vi "TSM Relay Control.vi"(0 "Relay TSM in":T1, 2 "Settling Time (s)":dbl, 5 "Relay Action":T3=21 items=["Open Relay"=20, "Close Relay"=21], 11 "error in":errorcluster) -> (15 "error out":errorcluster)   [LabVIEW 2020]
doc: "Performs the specified relay action on all specified relays."
uses:
  <vilib>/NI_TestStand_SemiconductorModule/NI_TestStand_Semiconductor_Module.lvlibp/1abvi3w/instr.lib/niSwitch/niswitch.llb/niSwitch Relay Action.ctl
  Pin Map/TSM Relay.ctl
  <vilib>/NI_TestStand_SemiconductorModule/NI_TestStand_Semiconductor_Module.lvlibp/PinMap/General/SemiconductorModuleContext.ctl
  <vilib>/NI_TestStand_SemiconductorModule/NI_TestStand_Semiconductor_Module.lvlibp/PinMap/Relay Driver/ControlRelaysSingleAction.vi
  <vilib>/NI_TestStand_SemiconductorModule/NI_TestStand_Semiconductor_Module.lvlibp
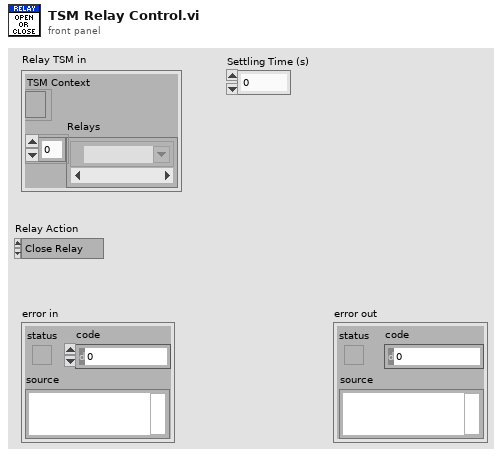
[diagram p1: front panel]
types:
  T1 = typedef "TSM Relay.ctl" = cluster{"TSM Context":T2, "Relays":tag[]}
  T2 = typedef "NI_TestStand_Semiconductor_Module.lvlibp/SemiconductorModuleContext.ctl" = refnum<k7>
  T3 = typedef "NI_TestStand_Semiconductor_Module.lvlibp/niSwitch Relay Action.ctl" = i32
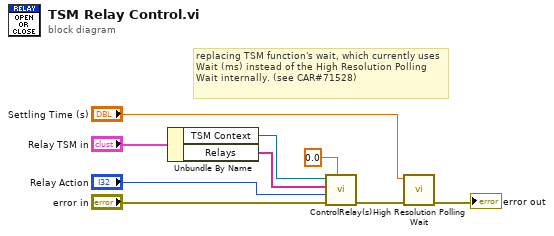
[diagram p0: block diagram]
diagram:
  # "replacing TSM function's wait, which currently uses Wait (ms) instead of the High Resolution Polling Wait internally. (see CAR#71528)"
  n1 = Unbundle By Name("Relay TSM in") -> ("TSM Context"=w2:T2, "Relays"=w1:tag[])
  n2 = call-poly <vilib>:"ControlRelay(s).vi"("Wait (s)"=0.0, "error in (no error)"="error in", "Relay Action"="Relay Action", "Relays"=w1, "Semiconductor Module Context"=w2) -> ("error out"=w7:errorcluster)  [unwired: 5 in, 1 out]
  n3 = call <vilib>:"High Resolution Polling Wait.vi"("error in (no error)"=w7, "seconds to wait"="Settling Time (s)") -> ("error out"=→"error out":errorcluster)  [unwired: 9 in]
